vi "Get Config File Location.vi"(8 "error in (no error)":errorcluster, 11 "Configuration File Path":path) -> (0 "error out":errorcluster, 3 "dup path":path)   [LabVIEW 2020, in "Execution UI.lvclass"]
uses:
  Execution UI.lvclass
  <vilib>/Utility/sysdir.llb/System Directory Type.ctl
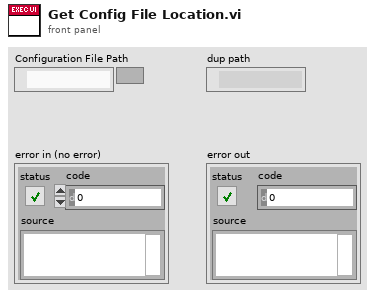
[diagram p1: front panel]
types:
  T1 = typedef "System Directory Type.ctl" = i32
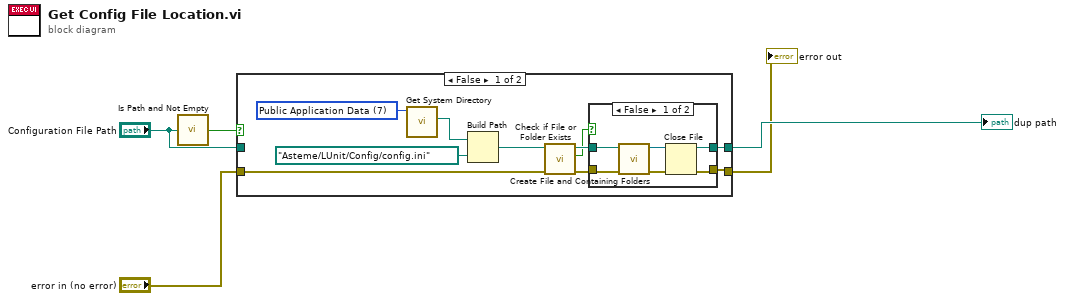
[diagram p0: block diagram]
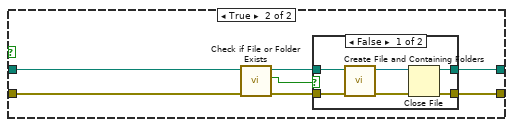
[diagram p3: hidden frame]
diagram:
  n1 = call <vilib>:"Is Path and Not Empty.vi"("path"="Configuration File Path") -> ("Is Path and Not Empty?"=w3:bool)  [unwired: 4 in]
  n2 = case shown="False" w3 {
    tunnel: [w12 w26] -> w1
    tunnel: "error in (no error)" -> [w7 w28]
    tunnel: [w11 w27] -> w5
    tunnel: "Configuration File Path" -> [_ w30]
    frame False {
      w13 = T1 7 items=["User Home"=0, "User Desktop"=1, "User Documents"=2, "User Application Data"=3, "User Preferences"=4, "User Temporary"=5, "Public Documents"=6, "Public Application Data"=7, "Public Preferences"=8, "Public Cache"=13, "System Core Libraries"=9, "System Installed Libraries"=10, "Application Files"=11, "Boot Volume Root"=12] ("system directory type")
      n3 = call <vilib>:"Get System Directory.vi"("system directory type"=w13) -> ("system directory"=w15:path)  [unwired: 10 in]
      n4 = Build Path(base path=w15, name or relative path=path "Asteme/LUnit/Config/config.ini") -> (appended path=w10:path)
      n5 = call <vilib>:"Check if File or Folder Exists.vi"("error in (no error)"=w7, "path"=w10) -> ("error out"=w8:errorcluster, "file or folder exists?"=w6:bool, "dup path"=w9:path)  [unwired: 7 in]
      n6 = case shown="False" w6 {
        tunnel: [w19 w22] -> w12
        tunnel: [w18 w23] -> w11
        tunnel: w9 -> [w17 w23]
        tunnel: w8 -> [w16 w22]
        frame False {
          n7 = call <vilib>:"Create File and Containing Folders.vi"("error in (no error)"=w16, "file path"=w17) -> ("error out"=w20:errorcluster, "refnum out"=w21:refnum<file>)  [unwired: 8 in]
          n8 = Close File(refnum=w21, error in=w20) -> (path=w18:path, error out=w19:errorcluster)
        }
        frame True {
        }
      }
    }
    frame True {
      n9 = call <vilib>:"Check if File or Folder Exists.vi"("error in (no error)"=w28, "path"=w30) -> ("error out"=w25:errorcluster, "file or folder exists?"=w24:bool, "dup path"=w29:path)  [unwired: 7 in]
      n10 = case shown="False" w24 {
        tunnel: w29 -> [w36 w38]
        tunnel: [w34 w38] -> w27
        tunnel: [w33 w37] -> w26
        tunnel: w25 -> [w31 w37]
        frame False {
          n11 = call <vilib>:"Create File and Containing Folders.vi"("error in (no error)"=w31, "file path"=w36) -> ("error out"=w32:errorcluster, "refnum out"=w35:refnum<file>)  [unwired: 8 in]
          n12 = Close File(refnum=w35, error in=w32) -> (path=w34:path, error out=w33:errorcluster)
        }
        frame True {
        }
      }
    }
  }
  "dup path" <- w5
  "error out" <- w1
